vi "SVFA Map Frequency to Order.vi"(10 "speed [RPM]":dbl=3600.0 min=0.0 step=1.0, 11 "frequency [Hz]":dbl=60.0 min=0.0 step=1.0) -> (3 "order":dbl=nan)   [LabVIEW 2017]
doc: "Use this VI to convert a frequency power spectrum to an order power spectrum. Use this VI to convert power spectrum results from constant-speed applications."
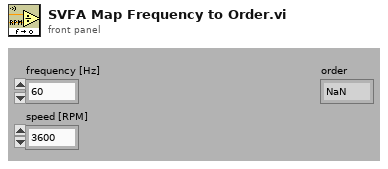
[diagram p1: front panel]
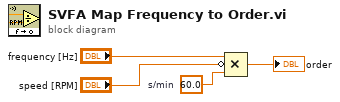
[diagram p0: block diagram]
diagram:
  w4 = 60.0  # s/min
  n1 = Compound Arithmetic op=MULTIPLY("frequency [Hz]", invert "speed [RPM]", w4) -> (→"order":dbl)
